vi "Solve Band Linear Equations.vi"   [LabVIEW 2020, in "NI_AALPro.lvlib"]
doc: "Computes the solution to the system of linear equations AX=Y with a band coefficient matrix A and single or multiple right-hand sides Y."
uses:
  <vilib>/Analysis/NI_AALPro.lvlib
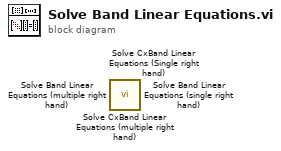
[diagram p0: block diagram]
diagram:
  n1 = call <vilib>:"Solve CxBand Linear Equations (multiple right hand).vi"() -> ()  [unwired: 10 in, 2 out]
  n2 = call <vilib>:"Solve CxBand Linear Equations (Single right hand).vi"() -> ()  [unwired: 10 in, 2 out]
  n3 = call <vilib>:"Solve Band Linear Equations (multiple right hand).vi"() -> ()  [unwired: 10 in, 2 out]
  n4 = call <vilib>:"Solve Band Linear Equations (single right hand).vi"() -> ()  [unwired: 10 in, 2 out]
